vi "ReadTag.vi"(7 "Slave Address (7-bit)":u8, 8 "error in (no error)":errorcluster, 9 "Timeout (ms)":i32=1000, 10 "DI Ref Out":T9, 11 "I2C Ref Out in":T1) -> (0 "error out":errorcluster, 1 "UID":string, 2 "DIO Ref Out out":T9, 3 "I2C Ref Out out":T1, 4 "Bytes Read":u8[](array[numeric]) format="%02x", 5 "# of tags":u8, 6 "Timeout READ":bool)   [LabVIEW 2015]
uses:
  <vilib>/myRIO/Instrument Drivers/Onboard IO/DIO/typedefs/DIO Reference.ctl
  <vilib>/myRIO/Common/Instrument Driver Framework/Utilities/typedefs/myRIO Generic Hardware Reference.ctl
  <vilib>/myRIO/Common/Instrument Driver Framework/Utilities/typedefs/Hardware Version Enum.ctl
  <vilib>/myRIO/Common/Instrument Driver Framework/Utilities/typedefs/myRIO v1.0 Reference.ctl
  <vilib>/myRIO/Common/Instrument Driver Framework/Utilities/typedefs/Generic FPGA Reference.ctl
  <vilib>/myRIO/Common/Instrument Driver Framework/myRIO v1.0/DIO/typedefs/DIO Channels List.ctl
  <vilib>/myRIO/Common/Instrument Driver Framework/myRIO v1.0/DIO/typedefs/DIO Channels Enum.ctl
  <vilib>/myRIO/Instrument Drivers/Onboard IO/I2C/typedefs/I2C Reference.ctl
  <vilib>/myRIO/Common/Instrument Driver Framework/myRIO v1.0/I2C/typedefs/I2C Channels Enum.ctl
  <vilib>/myRIO/Instrument Drivers/Onboard IO/I2C/typedefs/I2C Configuration.ctl
  <vilib>/myRIO/Instrument Drivers/Onboard IO/I2C/typedefs/I2C Transfer Rate.ctl
  <vilib>/Utility/error.llb/Error Cluster From Error Code.vi
  <vilib>/myRIO/Common/Instrument Driver Framework/myRIO v1.0/I2C/vis/myRIO v1.0 Read I2C.vi
  <vilib>/myRIO/Instrument Drivers/Onboard IO/I2C/I2C.lvlib
  <vilib>/myRIO/Instrument Drivers/Onboard IO/DIO/DIO.lvlib
panel:
  out "ACK Read CMD":bool
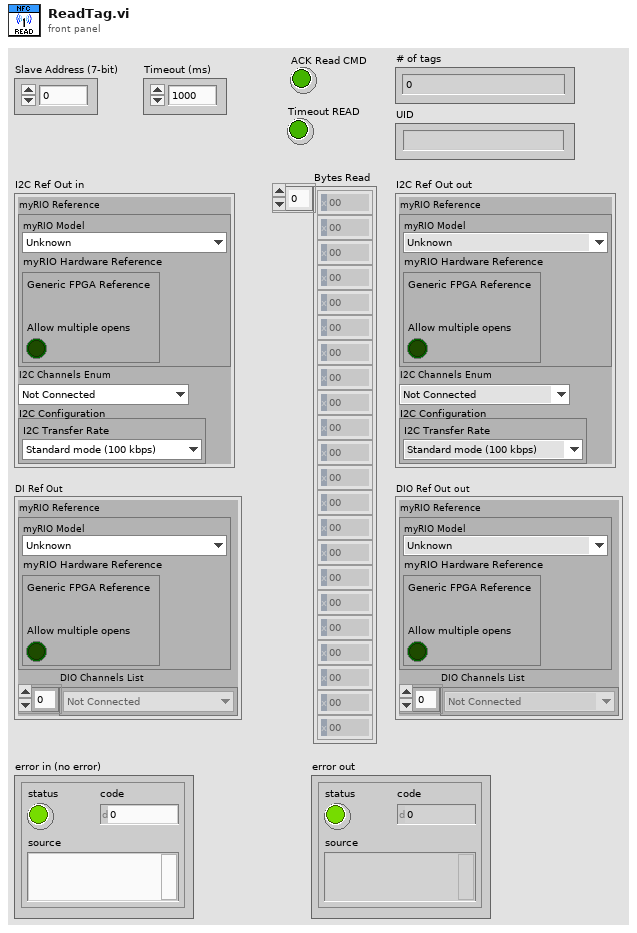
[diagram p1: front panel]
types:
  T1 = typedef "I2C.lvlib/I2C Reference.ctl" = cluster{"myRIO Reference":T2, "I2C Channels Enum":T6, "I2C Configuration":T7}
  T2 = typedef "myRIO Generic Hardware Reference.ctl" = cluster{"myRIO Model":T3, "myRIO Hardware Reference":T4}
  T3 = typedef "Hardware Version Enum.ctl" = enum16{"Unknown", "myRIO-1900", "myRIO-1950", "roboRIO"}
  T4 = typedef "myRIO v1.0 Reference.ctl" = cluster{"Generic FPGA Reference":T5, "Allow multiple opens":bool}
  T5 = typedef "Generic FPGA Reference.ctl" = refnum<k20>
  T6 = typedef "I2C Channels Enum.ctl" = enum16{"Not Connected", "A/I2C", "B/I2C", "I2C/I2C"}
  T7 = typedef "I2C.lvlib/I2C Configuration.ctl" = cluster{"I2C Transfer Rate":T8}
  T8 = typedef "I2C.lvlib/I2C Transfer Rate.ctl" = enum16{"Standard mode (100 kbps)", "Fast mode (400 kbps)"}
  T9 = typedef "DIO.lvlib/DIO Reference.ctl" = cluster{"myRIO Reference":T2, "DIO Channels List":T10}
  T10 = typedef "DIO Channels List.ctl" = T11[]
  T11 = typedef "DIO Channels Enum.ctl" = enum16{"Not Connected", "C/DIO0", "C/DIO1", "C/DIO2", "C/DIO3", "C/DIO4", "C/DIO5", "C/DIO6", "C/DIO7", "A/DIO0", "A/DIO1", "A/DIO2", "A/DIO3", "A/DIO4", "A/DIO5", "A/DIO6", "A/DIO7", "A/DIO8", "A/DIO9", "A/DIO10", "A/DIO11", "A/DIO12", "A/DIO13", "A/DIO14", "A/DIO15", "B/DIO0", "B/DIO1", "B/DIO2", "B/DIO3", "B/DIO4", "B/DIO5", "B/DIO6", "B/DIO7", "B/DIO8", "B/DIO9", "B/DIO10", "B/DIO11", "B/DIO12", "B/DIO13", "B/DIO14", "B/DIO15", "LED0", "LED1", "LED2", "LED3", "Button0", "DIO/DIO0", "DIO/DIO1", "DIO/DIO2", "DIO/DIO3", "DIO/DIO4", "DIO/DIO5", "DIO/DIO6", "DIO/DIO7", "DIO/DIO8", "DIO/DIO9", "SPI/CS0", "SPI/CS1", "SPI/CS2", "SPI/CS3", "LED RADIO (Green)", "LED RADIO (Red)", "LED COMM (Green)", "LED COMM (Red)", "LED MODE (Green)", "LED MODE (Red)"}
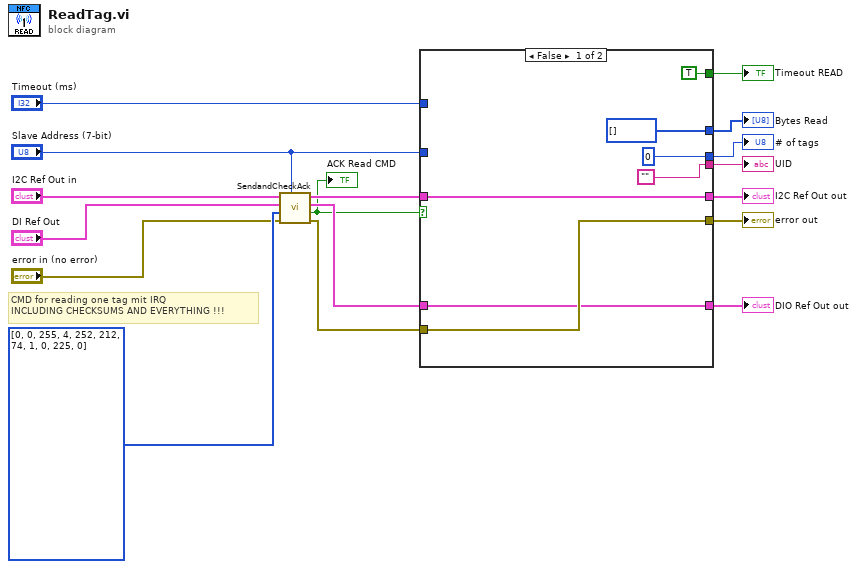
[diagram p0: block diagram]
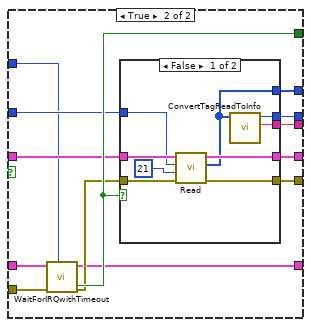
[diagram p2: hidden frame]
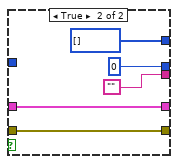
[diagram p3: hidden frame]
diagram:
  # "CMD for reading one tag mit IRQ\nINCLUDING CHECKSUMS AND EVERYTHING !!!"
  n1 = call "SendandCheckAck.vi"("Slave Address (7-bit)"="Slave Address (7-bit)", "error in (no error)"="error in (no error)", "bytes to send"=u8[] [0, 0, 255, 4, 252, 212, 74, 1, 0, 225, 0], "DI Ref In"="DI Ref Out", "I2C Ref In"="I2C Ref Out in") -> ("error out"=w14:errorcluster, "ACK?"=w2:bool, "DI Ref Out"=w12:T9, "I2C Ref Out"=w11:T1)  [unwired: 1 in, 2 out]
  "ACK Read CMD" <- w2
  n2 = case shown="False" w2 {
    tunnel: [TRUE ("Timed out?") w37] -> w15
    tunnel: w14 -> [w19 w35]
    tunnel: "Slave Address (7-bit)" -> [_ w34]
    tunnel: w12 -> [w18 w33]
    tunnel: w11 -> [w20 w32]
    tunnel: [w18 w31] -> w8
    tunnel: [w19 w30] -> w7
    tunnel: [w20 w29] -> w6
    tunnel: [u8[] [] ("Bytes Read") w28] -> w5
    tunnel: [u8 0 ("# of tags") w27] -> w4
    tunnel: ["" w26] -> w3
    tunnel: "Timeout (ms)" -> [_ w25]
    frame False {
    }
    frame True {
      n3 = call "WaitForIRQwithTimeout.vi"("Timeout (ms)"=w25, "error in (no error)"=w35, "DIO Ref Out in"=w33) -> ("error out"=w36:errorcluster, "DIO Ref Out out"=w31:T9, "Timed out?"=w37:bool)  [unwired: 6 in]
      n4 = case shown="False" w37 {
        tunnel: [w45 w51] -> w29
        tunnel: [w44 w50] -> w30
        tunnel: w32 -> [w43 w51]
        tunnel: w34 -> [w42 _]
        tunnel: w36 -> [w41 w50]
        tunnel: [w40 u8[] [] ("Bytes Read")] -> w28
        tunnel: [w39 u8 0 ("# of tags")] -> w27
        tunnel: [w38 ""] -> w26
        frame False {
          n5 = call <vilib>:"Read.vi"("error in (no error)"=w41, "Byte Count"=u32 21, "Slave Address (7-bit)"=w42, "I2C Ref In"=w43) -> ("error out"=w44:errorcluster, "Bytes Read"=w40:u8[], "I2C Ref Out"=w45:T1)  [unwired: 4 in]
          n6 = call "ConvertTagReadToInfo.vi"("Bytes Read"=w40) -> ("UID"=w38:string, "# of tags"=w39:u8)  [unwired: 9 in]
        }
        frame True {
        }
      }
    }
  }
  "Timeout READ" <- w15
  "DIO Ref Out out" <- w8
  "error out" <- w7
  "I2C Ref Out out" <- w6
  "Bytes Read" <- w5
  "# of tags" <- w4
  "UID" <- w3
